vi "Mercury_GoToField.vi"(8 "error in":errorcluster, 10 "persistent mode":bool=TRUE, 11 "Mercury Targets":T1={"Target Field (T)"=0.1, "Target Field Rate (T/min)"=0.1}) -> (0 "error out":errorcluster)   [LabVIEW 2016, in "Instrument.Oxford1820.lvclass"]
doc: "Use this VI to remotely interact with the Oxford Mercury power supply through \"Oxford-1820-Main.vi\", which MUST also be running."
uses:
  Instrument.Oxford1820.lvclass
  Typedefs/Targets.ctl
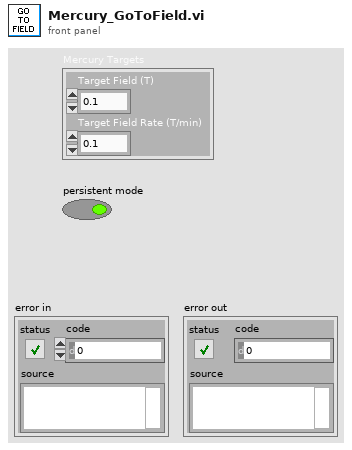
[diagram p1: front panel]
types:
  T1 = typedef "Instrument.Oxford1820.lvclass/Targets.ctl" = cluster{"Target Field (T)":dbl, "Target Field Rate (T/min)":dbl}
  T2 = typedef "Instrument.Oxford1820.lvclass/Status.ctl" = cluster{"Magnet Field":dbl, "PS Field":dbl, "Target Field":dbl, "Target Field Rate":dbl, "Voltage":dbl, "Current":dbl, "Switch":bool, "Mercury State":string}
  T3 = typedef "Instrument.Oxford1820.lvclass/Actions.ctl" = cluster{"Hold":bool, "Clamp":bool, "To Set":bool, "To Zero":bool, "Send to IPS":bool, "PS Heat":bool, "Lambda":bool}
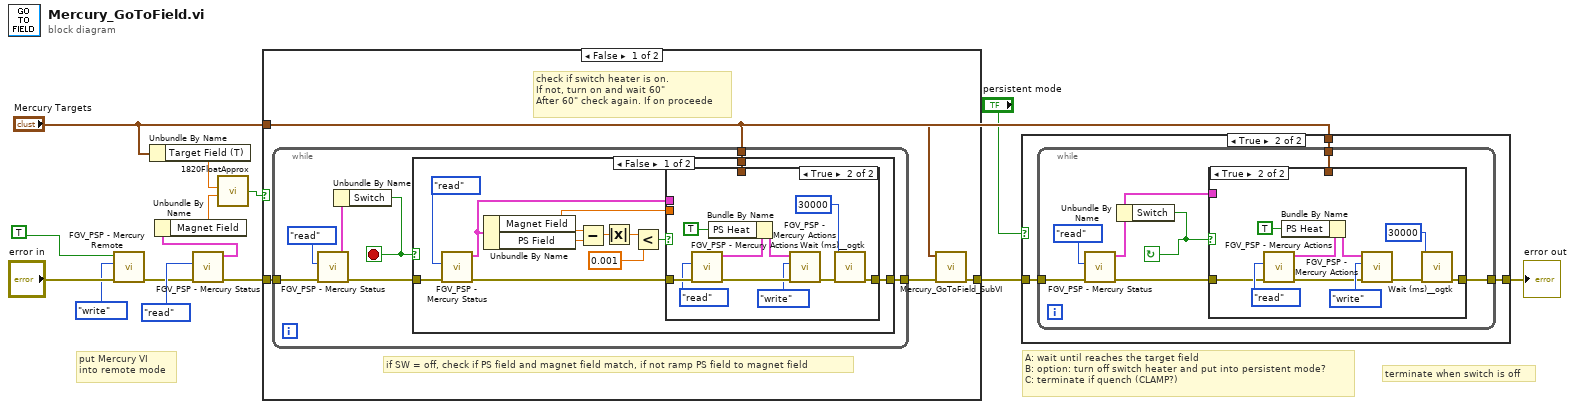
[diagram p0: block diagram]
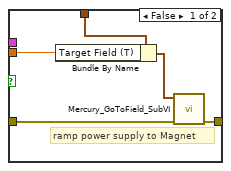
[diagram p2: hidden frame]
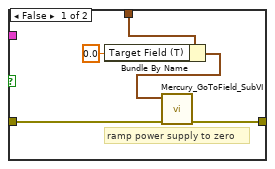
[diagram p6: hidden frame]
diagram:
  # "terminate when switch is off"
  # "A: wait until reaches the target field\nB: option: turn off switch heater and put into persistent mode?\nC: terminate if quench (CLAMP?)"
  # "put Mercury VI\ninto remote mode"
  n1 = call "FGV_PSP - Mercury Remote.vi"("error in"="error in", "Function"=enum16{"write", "read"}."write", "Remote"=TRUE ("Mercury Remote")) -> ("error out"=w3:errorcluster)  [unwired: 3 in, 1 out]
  n2 = Unbundle By Name("Mercury Targets") -> ("Target Field (T)"=w11:dbl)
  n3 = call "FGV_PSP - Mercury Status.vi"("error in"=w3, "Function"=enum16{"write", "read"}."read") -> ("error out"=w6:errorcluster, "Status"=w7:T2)  [unwired: 4 in]
  n4 = Unbundle By Name(w7) -> ("Magnet Field"=w9:dbl)
  n5 = call "1820FloatApprox.vi"("y"=w9, "x"=w11) -> ("x ~ y?"=w10:bool)  [unwired: 2 in]
  n6 = case shown="False" w10 {
    tunnel: w6 -> [w18 w54]
    tunnel: [w16 w54] -> w14
    tunnel: "Mercury Targets" -> [w15 _]
    frame False {
      # "if SW = off, check if PS field and magnet field match, if not ramp PS field to magnet field"
      # "check if switch heater is on.\nIf not, turn on and wait 60\"\nAfter 60\" check again. If on proceede"
      n7 = while {
        tunnel: [w24] -> w17
        tunnel: w18 -> [w20]
        tunnel: w15 -> [w23]
        stop <- w25 stop-if-true
        n8 = call "FGV_PSP - Mercury Status.vi"("error in"=w20, "Function"=enum16{"write", "read"}."read") -> ("error out"=w19:errorcluster, "Status"=w21:T2)  [unwired: 4 in]
        n9 = Unbundle By Name(w21) -> ("Switch"=w25:bool)
        n10 = case shown="False" w25 {
          tunnel: w19 -> [w28 w53]
          tunnel: [w37 w53] -> w24
          tunnel: w23 -> [w31 _]
          frame False {
            n11 = call "FGV_PSP - Mercury Status.vi"("error in"=w28, "Function"=enum16{"write", "read"}."read") -> ("error out"=w27:errorcluster, "Status"=w26:T2)  [unwired: 4 in]
            n12 = Unbundle By Name(w26) -> ("Magnet Field"=w30:dbl, "PS Field"=w36:dbl)
            n13 = Subtract(x=w30, y=w36) -> (x-y=w35:dbl)
            n14 = Absolute Value(x=w35) -> (abs(x)=w34:dbl)
            n15 = Less?(x=w34, y=0.001) -> (x < y?=w32:bool)
            n16 = case shown="True" w32 {
              tunnel: [w41 w51] -> w37
              tunnel: w27 -> [w42 w49]
              tunnel: w31 -> [w40 _]
              tunnel: w30 -> [w39 _]
              tunnel: w26 -> [_ _]
              frame False {
                # "ramp power supply to Magnet"
                n17 = Bundle By Name(cluster=w40, "Target Field (T)"=w39) -> (w38:T1)
                n18 = call "Mercury_GoToField_SubVI.vi"("error in (no error)"=w42, "Targets"=w38) -> ("error out"=w41:errorcluster)  [unwired: 9 in]
              }
              frame True {
                n19 = call "FGV_PSP - Mercury Actions.vi"("error in"=w49, "Function"=enum16{"write", "read"}."read") -> ("error out"=w47:errorcluster, "Actions"=w44:T3)  [unwired: 4 in]
                n20 = Bundle By Name(cluster=w44, "PS Heat"=TRUE ("Send to IPS")) -> (w45:T3)
                n21 = call "FGV_PSP - Mercury Actions.vi"("error in"=w47, "Function"=enum16{"write", "read"}."write", "Actions"=w45) -> ("error out"=w43:errorcluster)  [unwired: 3 in, 1 out]
                n22 = call <userlib>:"Wait (ms)__ogtk.vi"("error in (no error)"=w43, "milliseconds to wait"=u32 30000) -> ("error out"=w51:errorcluster)  [unwired: 8 in, 1 out]
              }
            }
          }
          frame True {
          }
        }
      }
      n23 = call "Mercury_GoToField_SubVI.vi"("error in (no error)"=w17, "Targets"=w15) -> ("error out"=w16:errorcluster)  [unwired: 9 in]
    }
    frame True {
      # "if magnet is already at target field skip ramping up leads. just\ncheck if in persistent mode."
    }
  }
  n24 = case shown="True" "persistent mode" {
    tunnel: w14 -> [w55 w58]
    tunnel: "Mercury Targets" -> [_ w57]
    tunnel: [w55 w56] -> w13
    frame False {
    }
    frame True {
      n25 = while {
        tunnel: [w65] -> w56
        tunnel: w58 -> [w59]
        tunnel: w57 -> [w64]
        stop <- w63 continue-if-true
        n26 = call "FGV_PSP - Mercury Status.vi"("error in"=w59, "Function"=enum16{"write", "read"}."read") -> ("error out"=w60:errorcluster, "Status"=w61:T2)  [unwired: 4 in]
        n27 = Unbundle By Name(w61) -> ("Switch"=w63:bool)
        n28 = case shown="True" w63 {
          tunnel: [w70 w79] -> w65
          tunnel: w64 -> [w69 _]
          tunnel: w60 -> [w66 w72]
          tunnel: w61 -> [_ _]
          frame False {
            # "ramp power supply to zero"
            n29 = Bundle By Name(cluster=w69, "Target Field (T)"=0.0) -> (w68:T1)
            n30 = call "Mercury_GoToField_SubVI.vi"("error in (no error)"=w66, "Targets"=w68) -> ("error out"=w70:errorcluster)  [unwired: 9 in]
          }
          frame True {
            n31 = call "FGV_PSP - Mercury Actions.vi"("error in"=w72, "Function"=enum16{"write", "read"}."read") -> ("error out"=w71:errorcluster, "Actions"=w75:T3)  [unwired: 4 in]
            n32 = Bundle By Name(cluster=w75, "PS Heat"=TRUE ("Send to IPS")) -> (w74:T3)
            n33 = call "FGV_PSP - Mercury Actions.vi"("error in"=w71, "Function"=enum16{"write", "read"}."write", "Actions"=w74) -> ("error out"=w76:errorcluster)  [unwired: 3 in, 1 out]
            n34 = call <userlib>:"Wait (ms)__ogtk.vi"("error in (no error)"=w76, "milliseconds to wait"=u32 30000) -> ("error out"=w79:errorcluster)  [unwired: 8 in, 1 out]
          }
        }
      }
    }
  }
  "error out" <- w13
